vi "CALC_CUST_DEF_M.vi"(0 "VISA IN":refnum<visa-resource-name>, 1 "Measurement Name":string, 2 "Measurement Type":string, 3 "Measurement Parameter":string, 5 "error in":errorcluster, 7 "Channel":i32) -> (14 "VISA Out":refnum<visa-resource-name>, 16 "Meas":string, 17 "Filename":string, 19 "error out":errorcluster)   [LabVIEW 2018, in "PNA-X.lvlib"]
doc: "CALCulate<cnum>:CUSTom:DEFine <Mname>, <type> [,param] \n(Write-only) Creates a custom measurement. The custom measurement is not automatically \ndisplayed. You must also do the following: \nUse DISP:WIND:STATe to create a window if it doesn't already exist.� \nUse DISP:WIND:TRAC:FEED to display the measurement \nSelect the measurement (CALC:PAR:SEL) before making additional settings. \nSee an example using this command to create a VMC and SMC measurement \nParameters \n<cnum> Any existing channel number. If unspecified, value is set to 1. \n<Mname> Name of the measurement. Any non-empty, unique string, enclosed in quotes. \n<type> String. The type of custom measurement. Choose from: \n\"Vector Mixer/Converter\" \n\"Scalar Mixer/Converter\" \nThese arguments are new with PNA release 6.0. The old arguments are still \nsupported. \n[param] String. Optional parameter specifies the measurement parameter to create. \n1492\n\nType Valid Parameters: \nVector Mixer/Converter \"S11\" \n\"VC21\" \n\"S22\" \nScalar Mixer/Converter \"S11\" \n\"SC21\" \n\"SC12\" \n\"S22\" \n\"Ipwr\" \n\"RevIPwr\" \n\"Opwr\" \n\"RevOPwr\" \nExamples CALC2:CUST:DEF 'My VC21', 'Vector Mixer/Converter','S22' \nQuery Syntax Not applicable \nOverlapped? No \nDefault Not applicable"
uses:
  PNA-X.lvlib
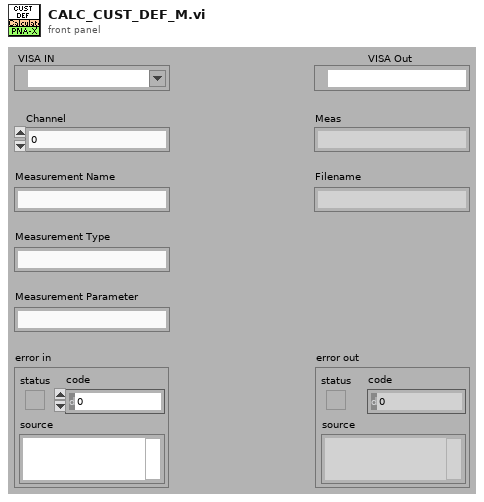
[diagram p1: front panel]
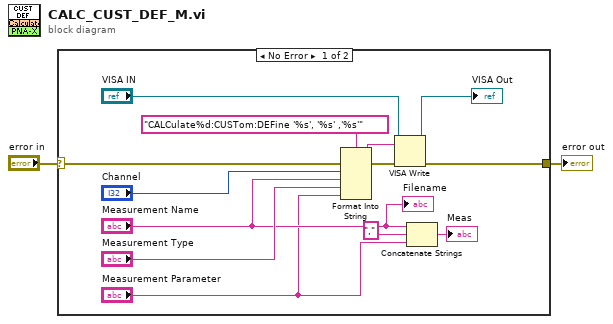
[diagram p0: block diagram]
diagram:
  n1 = case shown="No Error" "error in" {
    selector: "error in" -> [w15 w16]
    tunnel: [w10 w16] -> w1
    frame No Error {
      n2 = Format Into String(format string="CALCulate%d:CUSTom:DEFine '%s', '%s' ,'%s'" ("Cmdline"), error in=w15, "Channel", "Measurement Name", "Measurement Type", "Measurement Parameter") -> (resulting string=w13:string, error out=w14:errorcluster)  [unwired: 1 in]
      n3 = VISA Write(VISA resource name="VISA IN", write buffer=w13, error in (no error)=w14) -> (VISA resource name out=→"VISA Out":refnum<visa-resource-name>, error out=w10:errorcluster)  [unwired: 1 out]
      n4 = Concatenate Strings("Measurement Name", "," ("string"), "Measurement Parameter") -> (→"Meas":string)
      "Filename" <- "Measurement Name"
    }
    frame Error {
    }
  }
  "error out" <- w1
